vi "SLSC Add Property Section.vi"(6 "enums":T1[](array[typedef]), 8 "error in (no error)":errorcluster, 9 "Physical Channel":string, 10 "properties":T3[](array[typedef]), 11 "Parent Ref in":T2 format="%.0x") -> (0 "error out":errorcluster, 3 "Parent Ref out":T2 format="%.0x")   [LabVIEW 2019, in "SLSC EDS System Explorer.lvlib"]
uses:
  System Explorer/SLSC EDS System Explorer.lvlib
  SLSC EDS API/JSON parsing/property.ctl
  <vilib>/NI VeriStand/Custom Device API/Custom Device Item Ref.ctl
  SLSC EDS API/JSON parsing/enum.ctl
  Shared/Constants.vi
  Shared/SLSC EDS Shared.lvlib
  SLSC CD System Explorer.lvlib
  <vilib>/NI VeriStand/Custom Device API/Custom Device API.lvlib
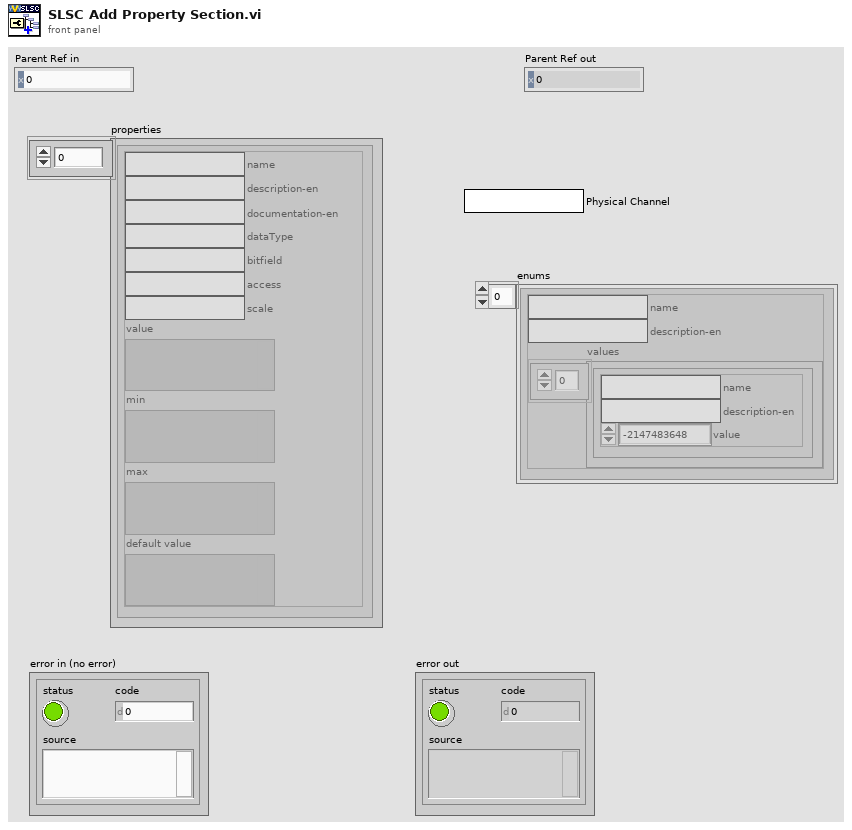
[diagram p1: front panel]
types:
  T1 = typedef "enum.ctl" = cluster{"name":string, "description-en":string, "values":cluster{"name":string, "description-en":string, "value":i32}[]}
  T2 = typedef "Custom Device API.lvlib/Custom Device Item Ref.ctl" = u64
  T3 = typedef "property.ctl" = cluster{"name":string, "description-en":string, "documentation-en":string, "dataType":string, "bitfield":string, "access":string, "scale":string, "value":variant, "min":variant, "max":variant, "default value":variant}
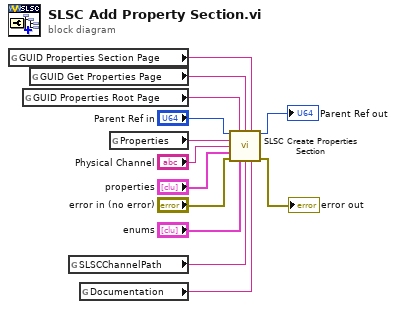
[diagram p0: block diagram]
diagram:
  n1 = global read "Constants.vi" "GUID Properties Section Page"() -> (w1:string)
  n2 = global read "Constants.vi" "GUID Properties Root Page"() -> (w11:string)
  n3 = global read "Constants.vi" "GUID Get Properties Page"() -> (w2:string)
  n4 = global read "Constants.vi" "SLSCChannelPath"() -> (w4:string)
  n5 = global read "Constants.vi" "Documentation"() -> (w3:string)
  n6 = global read "Constants.vi" "Properties"() -> (w10:string)
  n7 = call "SLSC Create Properties Section.vi"("Parent Ref in"="Parent Ref in", "GUID Properties Root Page"=w11, "GUID Get Properties Page"=w2, "GUID Set Properties Page"=w1, "Properties"=w10, "Physical Channel"="Physical Channel", "properties"="properties", "error in (no error)"="error in (no error)", "enums"="enums", "SLSCChannelPath"=w4, "Documentation"=w3) -> ("Parent Ref out"=→"Parent Ref out":T2, "error out"=→"error out":errorcluster)  [unwired: 3 in]
